vi "B Spoof Relative Wind.vi"(4 "Robot velocity":T1 {"East" format="%#_5g"}, 6 "Wind Speed":dbl, 7 "Wind Angle":T2 format="%05.1f", 8 "Velocity (3 array)":dbl[](array[numeric])) -> (0 "Apparent Wind\nSpeed":T3, 1 "Perceived Wind":cluster{"X Position":dbl, "Y Position":dbl}, 2 "Apparent Wind\nDirection":T4, 3 "Global Wind":cluster{"X Position":dbl, "Y Position":dbl}, 5 "Robot\nHeading":T2 format="%05.1f")   [LabVIEW 2011]
uses:
  2-Think/2 Typedefs/heading.ctl
  2-Think/2 Typedefs/apparent wind direction.ctl
  2-Think/2 Typedefs/apparent wind speed.ctl
  2-Think/2 Typedefs/Velocity.ctl
  <vilib>/Analysis/_algsub.llb/Real Vector Norm.vi
  <vilib>/Analysis/baseanly.llb/Real Dot Product.vi
  <vilib>/Analysis/NI_AALPro.lvlib
  <vilib>/Analysis/NI_AALBase.lvlib
panel:
  out "x*y":cluster{"X Position":dbl, "Y Position":dbl}
  out "Heading Out":T2 format="%05.1f"
  out "Heading unit\nvector":cluster{"X Position":dbl, "Y Position":dbl}
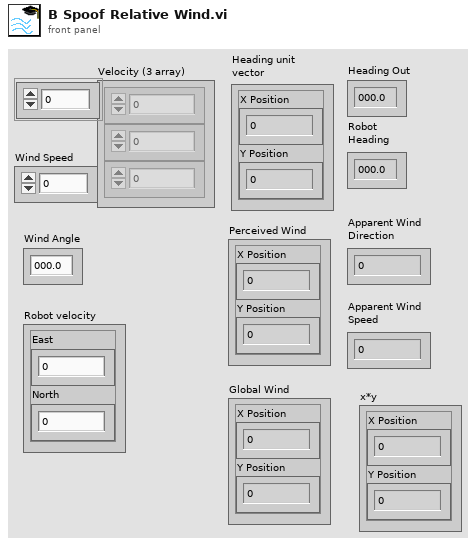
[diagram p1: front panel]
types:
  T1 = typedef "Velocity.ctl" = cluster{"East":dbl, "North":dbl}
  T2 = typedef "heading.ctl" = dbl
  T3 = typedef "apparent wind speed.ctl" = dbl
  T4 = typedef "apparent wind direction.ctl" = dbl
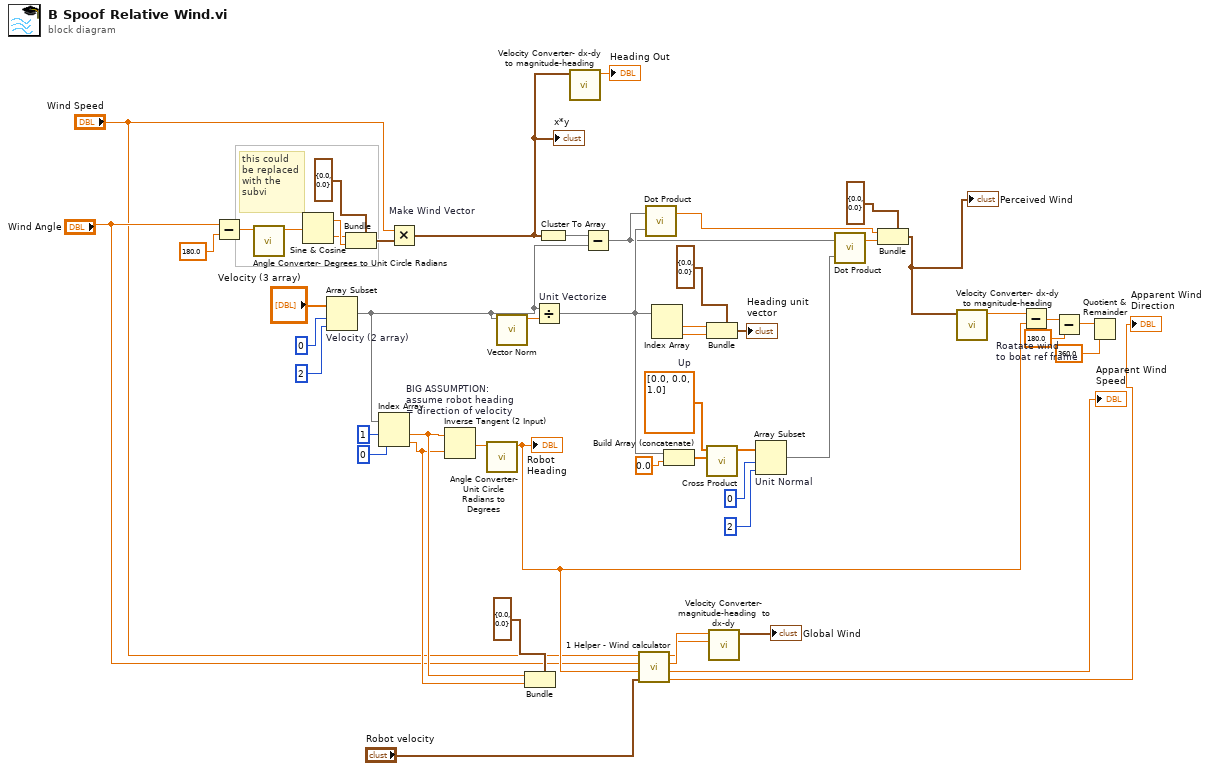
[diagram p0: block diagram]
diagram:
  w28 = dbl[] [0.0, 0.0, 1.0]  # Up
  # "this could\nbe replaced\nwith the\nsubvi"
  n1 = Subtract(x="Wind Angle", y=T2 180.0 ("Wind Angle 2")) -> (x-y=w26:T2)
  n2 = call "Angle Converter- Degrees to Unit Circle Radians.vi"("Angle in \nHeading \nFormat"=w26) -> ("Angle in \nUnit Circle\nRadians"=w27:dbl)  [unwired: 10 in]
  n3 = Sine & Cosine(0:w27) -> (1:w42:dbl, 2:w41:dbl)
  n4 = Array Subset "Velocity (2 array)"(array="Velocity (3 array)", index=0, length=2) -> (w23:dbl[])
  n5 = Bundle(cluster=cluster{"X Position":dbl, "Y Position":dbl} {"X Position"=0.0, "Y Position"=0.0} ("Robot Location"), "X Position"=w41, "Y Position"=w42) -> (w43:cluster{"X Position":dbl, "Y Position":dbl})
  n6 = Index Array(array=w23, index #1=1 ("index"), index #2=0 ("index")) -> (element #1=w12:dbl, element #2=w11:dbl)
  n7 = Multiply "Make Wind Vector"(x="Wind Speed", y=w43) -> (x*y=w15:cluster{"X Position":dbl, "Y Position":dbl})
  "x*y" <- w15
  n8 = Inverse Tangent (2 Input) "BIG ASSUMPTION:\nassume robot heading\n= direction of velocity"(1:w11, 2:w12) -> (0:w24:dbl)
  n9 = call "Angle Converter- Unit Circle Radians to Degrees.vi"("Angle in \nUnit Circle\nRadians"=w24) -> ("Angle in \nHeading \nFormat"=w10:T2)  [unwired: 10 in]
  "Robot\nHeading" <- w10
  n10 = call-poly <vilib>:"Vector Norm.vi"("Input Vector"=w23) -> ("norm"=w52:dbl)  [unwired: 9 in, 1 out]
  n11 = Bundle(cluster=cluster{"X Position":dbl, "Y Position":dbl} {"X Position"=0.0, "Y Position"=0.0} ("Robot Location"), "X Position"=w12, "Y Position"=w11) -> ()  [unwired: 1 out]
  n12 = Divide "Unit Vectorize"(x=w23, y=w52) -> (x/y=w37:dbl[])
  n13 = Cluster To Array(cluster=w15) -> (array=w49:dbl[])
  n14 = call "Velocity Converter- dx-dy to magnitude-heading.vi"("Vector In"=w15) -> ("Heading Out"=→"Heading Out":T2)  [unwired: 9 in, 1 out]
  n15 = Subtract(x=w49, y=w23) -> (x-y=w32:dbl[])
  n16 = call "1 Helper - Wind calculator.vi"("Robot Velocity"="Robot velocity", "Heading"=w10, "Absolute Wind Direction"="Wind Angle", "Absolute Wind Speed"="Wind Speed") -> ("Apparent Wind Direction"=→"Apparent Wind\nDirection":T2, "Apparent Wind Speed"=→"Apparent Wind\nSpeed":T3, "Absolute Wind Direction"=w5:T2, "Absolute Wind Speed"=w4:dbl)  [unwired: 4 in]
  n17 = call-poly <vilib>:"Dot Product.vi"("Y Vector"=w37, "X Vector"=w32) -> ("X * Y"=w51:dbl)  [unwired: 1 out]
  n18 = Index Array(array=w37) -> (element #1=w46:dbl, element #2=w47:dbl)  [unwired: 2 in]
  n19 = Build Array (concatenate)(w37, 0.0) -> (w29:dbl[])
  n20 = Bundle(cluster=cluster{"X Position":dbl, "Y Position":dbl} {"X Position"=0.0, "Y Position"=0.0} ("Robot Location"), "X Position"=w46, "Y Position"=w47) -> (→"Heading unit\nvector":cluster{"X Position":dbl, "Y Position":dbl})
  n21 = call <vilib>:"Cross Product.vi"("B Vector"=w29, "A Vector"=w28) -> ("Cross Product"=w33:dbl[])  [unwired: 8 in, 1 out]
  n22 = call "Velocity Converter- magnitude-heading  to dx-dy.vi"("Magnitude"=w4, "Heading"=w5) -> ("Vector Out"=→"Global Wind":T1)  [unwired: 9 in]
  n23 = Array Subset "Unit Normal"(array=w33, index=0, length=2) -> (w31:dbl[])
  n24 = call-poly <vilib>:"Dot Product.vi"("Y Vector"=w31, "X Vector"=w32) -> ("X * Y"=w30:dbl)  [unwired: 1 out]
  n25 = Bundle(cluster=cluster{"X Position":dbl, "Y Position":dbl} {"X Position"=0.0, "Y Position"=0.0} ("Perceived Wind"), "X Position"=w51, "Y Position"=w30) -> (w1:cluster{"X Position":dbl, "Y Position":dbl})
  "Perceived Wind" <- w1
  n26 = call "Velocity Converter- dx-dy to magnitude-heading.vi"("Vector In"=w1) -> ("Heading Out"=w18:T2)  [unwired: 9 in, 1 out]
  n27 = Subtract "Roatate wind\nto boat ref frame"(x=w18, y=w10) -> (x-y=w20:T2)
  n28 = Subtract(x=w20, y=T2 180.0) -> (x-y=w17:T2)
  n29 = Quotient & Remainder(x=w17, y=T2 360.0) -> ()  [unwired: 2 out]
